vi "SUSLab.vi"() -> ()   [LabVIEW 2020]
panel:
  in  "Numeric":dbl
  out "Xwy":dbl
  in  "Thin":dbl
  in  "Pn":dbl
  in  "F":dbl
  in  "Delay":u32=100
  out "U":dbl
  in  "stop":bool
  out "Wykers":dbl(graph)
  in  "U":dbl(knob) scale=0.0..100.0
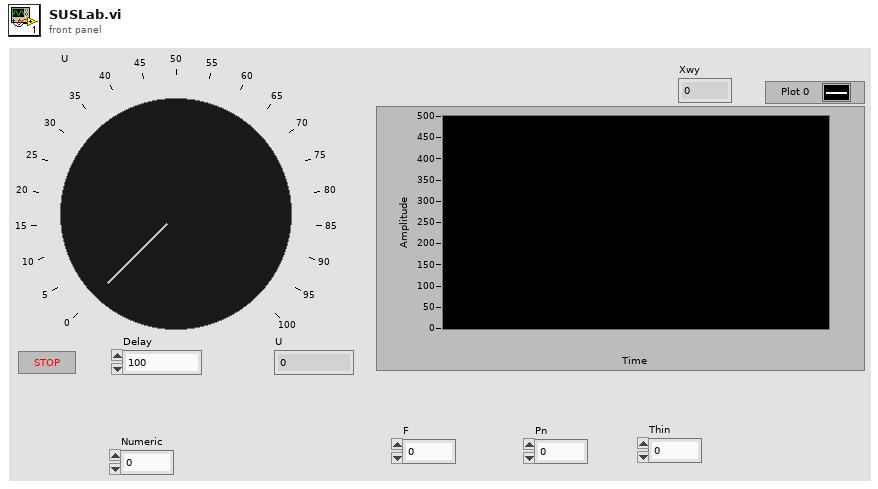
[diagram p1: front panel]
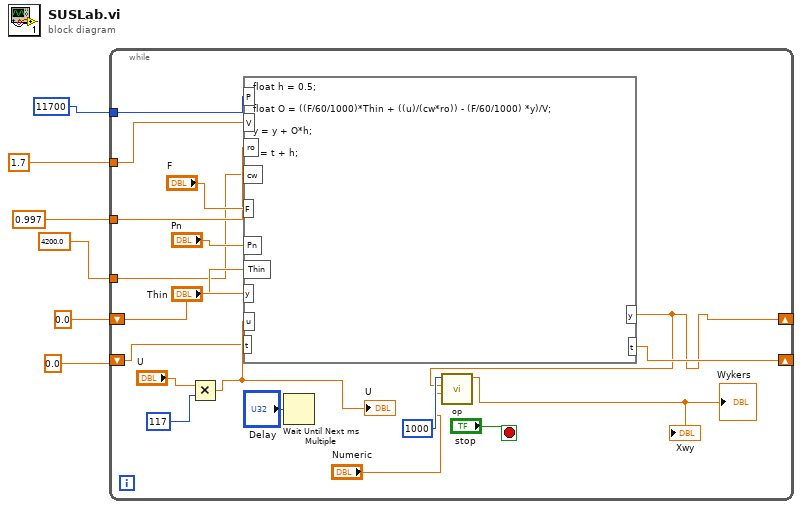
[diagram p0: block diagram]
diagram:
  n1 = while {
    shift-right: [w8] -> _
    shift-left: 0.0 -> [w25]
    tunnel: 1.7 ("V") -> [w16]
    tunnel: 0.997 ("ro") -> [w15]
    tunnel: 4200.0 ("cw") -> [w14]
    tunnel: 11700 -> [w13]
    shift-right: [w11] -> _
    shift-left: 0.0 -> [w12]
    stop <- "stop" stop-if-true
    n2 = Multiply(x="U", y=117) -> (x*y=w20:dbl)
    "U" <- w20
    n3 = formula code="float h = 0.5;\n\nfloat O = ((F/60/1000)*Thin + ((u)/(cw*ro)) - (F/60/1000) *y)/V;\n\ny = y + O*h;\n\nt = t + h;"("u"=w20, "y"=w25, "Thin"="Thin", "Pn"="Pn", "F"="F", "cw"=w14, "ro"=w15, "V"=w16, "P"=w13, "t"=w12) -> ("y"=w8:dbl, "t"=w11:dbl)
    n4 = Wait Until Next ms Multiple(millisecond multiple="Delay") -> ()  [unwired: 1 out]
    n5 = call "op.vi"("delay"="Numeric", "X0"=w8, "Xwe"=1000) -> ("Xwy"=→"Wykers" →"Xwy":dbl)  [unwired: 8 in]
  }
